vi "GoToNextCell.vi"(8 "Current Cell":T1, 9 "Column":i32, 10 "Row":i32, 11 "Board in":i32[][](array[numeric])) -> (0 "Current Cell":T1, 3 "Board out":i32[][](array[numeric]))   [LabVIEW 2023]
doc: "Go to next Cell by increasing Column and/or Row value for current Cell\n\nInputs\n- Board: Current Board Configuration\n- Row: Row of current Cell\n- Column: Column of current Cell\n- Current Cell: Row and Column of Current Cell\n\nOutputs\n- Board: Current Board Configuration\n- Current Cell: Row and Column of Current Cell"
uses:
  Controls/CurrentCell.ctl
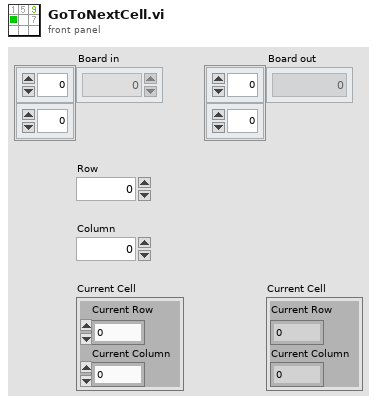
[diagram p1: front panel]
types:
  T1 = typedef "CurrentCell.ctl" = cluster{"Current Row":i32, "Current Column":i32}
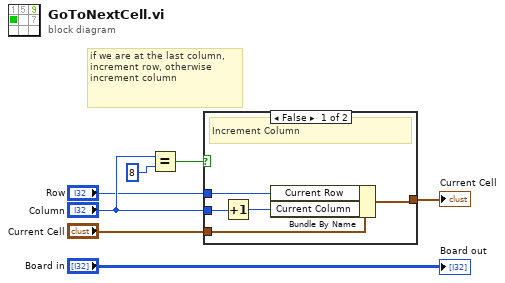
[diagram p0: block diagram]
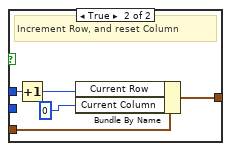
[diagram p2: hidden frame]
diagram:
  # "if we are at the last column, increment row, otherwise increment column"
  n1 = Equal?(x="Column", y=8) -> (x = y?=w2:bool)
  n2 = case shown="False" w2 {
    tunnel: "Row" -> [w12 w17]
    tunnel: "Column" -> [w11 _]
    tunnel: "Current Cell" -> [w9 w14]
    tunnel: [w8 w13] -> w6
    frame False {
      # "Increment Column"
      n3 = Increment(x=w11) -> (x+1=w10:i32)
      n4 = Bundle By Name(cluster=w9, "Current Row"=w12, "Current Column"=w10) -> (w8:T1)
    }
    frame True {
      # "Increment Row, and reset Column"
      n5 = Increment(x=w17) -> (x+1=w16:i32)
      n6 = Bundle By Name(cluster=w14, "Current Row"=w16, "Current Column"=0 ("element")) -> (w13:T1)
    }
  }
  "Current Cell" <- w6
  "Board out" <- "Board in"
